vi "sv_Get Function SubType String.vi"(4 "function subtype":T1 items=["Unscaled binary"=0, "Scaled voltage"=1, "Scaled engineering units"=2, "-"=10, "Value"=19, "DC"=11, "AC"=12, "RMS^2"=13, "RMS"=14, "Peak"=15, "Peak to peak"=16, "-"=20, "1/1 octave"=21, "1/3 octave"=22, "1/6 octave"=23, "1/12 octave"=24, "1/24 octave"=25, "-"=30, "Density"=31, "Magnitude"=32, "Phase"=33, "Real"=34, "Imaginary"=35, "Complex"=345, "Coherence"=36, "-"=90, "Unknown"=99]) -> (1 "function type string":string)   [LabVIEW 2017]
uses:
  <vilib>/addons/_NISVFA/_Shared subVIs/Controls/NI Function SubType.ctl
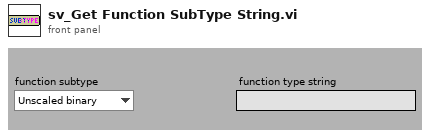
[diagram p1: front panel]
types:
  T1 = typedef "NI Function SubType.ctl" = u16
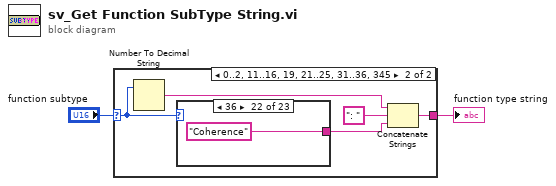
[diagram p0: block diagram]
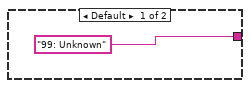
[diagram p2: hidden frame]
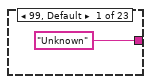
[diagram p3: hidden frame]
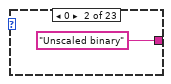
[diagram p4: hidden frame]
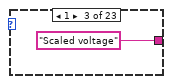
[diagram p5: hidden frame]
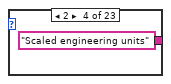
[diagram p6: hidden frame]
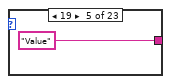
[diagram p7: hidden frame]
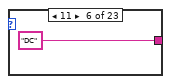
[diagram p8: hidden frame]
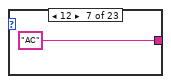
[diagram p9: hidden frame]
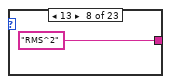
[diagram p10: hidden frame]
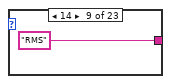
[diagram p11: hidden frame]
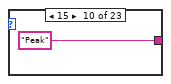
[diagram p12: hidden frame]
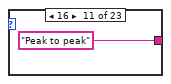
[diagram p13: hidden frame]
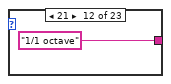
[diagram p14: hidden frame]
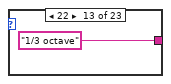
[diagram p15: hidden frame]
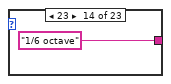
[diagram p16: hidden frame]
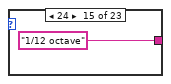
[diagram p17: hidden frame]
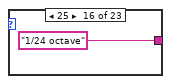
[diagram p18: hidden frame]
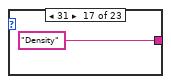
[diagram p19: hidden frame]
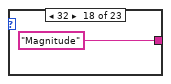
[diagram p20: hidden frame]
diagram:
  n1 = case shown="0..2, 11..16, 19, 21..25, 31..36, 345" "function subtype" {
    selector: "function subtype" -> [_ w6]
    tunnel: ["99: Unknown" ("String") w4] -> w1
    frame Default {
    }
    frame 0..2, 11..16, 19, 21..25, 31..36, 345 {
      n2 = Number To Decimal String(number=w6) -> (decimal integer string=w8:string)  [unwired: 1 in]
      n3 = case shown="36" w6 {
        tunnel: ["Unknown" ("String") "Unscaled binary" ("String") "Scaled voltage" ("String") "Scaled engineering units" ("String") "Value" ("String") "DC" ("String") "AC" ("String") "RMS^2" ("String") "RMS" ("String") "Peak" ("String") "Peak to peak" ("String") "1/1 octave" ("String") "1/3 octave" ("String") "1/6 octave" ("String") "1/12 octave" ("String") "1/24 octave" ("String") "Density" ("String") "Magnitude" ("String") "Phase" ("String") "Real" ("String") "Imaginary" ("String") "Coherence" ("String") "Complex" ("String")] -> w5
        frame 99, Default {
        }
        frame 0 {
        }
        frame 1 {
        }
        frame 2 {
        }
        frame 19 {
        }
        frame 11 {
        }
        frame 12 {
        }
        frame 13 {
        }
        frame 14 {
        }
        frame 15 {
        }
        frame 16 {
        }
        frame 21 {
        }
        frame 22 {
        }
        frame 23 {
        }
        frame 24 {
        }
        frame 25 {
        }
        frame 31 {
        }
        frame 32 {
        }
        frame 33 {
        }
        frame 34 {
        }
        frame 35 {
        }
        frame 36 {
        }
        frame 345 {
        }
      }
      n4 = Concatenate Strings(w8, ": " ("string"), w5) -> (w4:string)
    }
  }
  "function type string" <- w1
